vi "ScriptAllClasses.vi"(8 "error in (no error)":errorcluster, 11 "Application in":refnum<class "Application.lvclass">) -> (0 "error out":errorcluster, 3 "Application out":refnum<class "Application.lvclass">)   [LabVIEW 2020, in "Mermaid.lvlib" / "Application.lvclass"]
uses:
  Application.lvclass
  Application.lvclass/Application.ctl
  _Class/Class.lvclass
  _Interface/Interface.lvclass
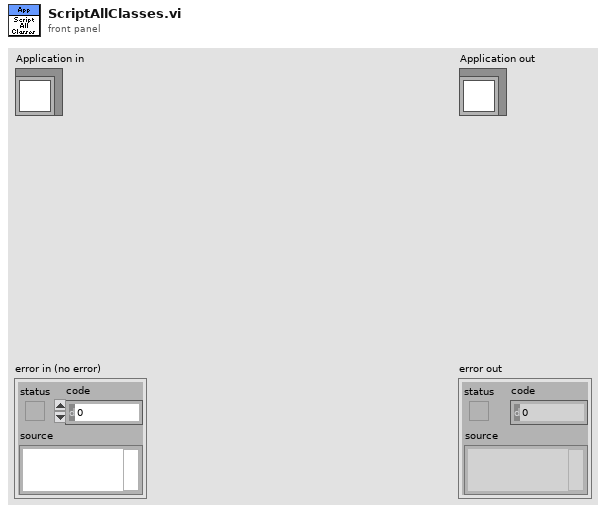
[diagram p1: front panel]
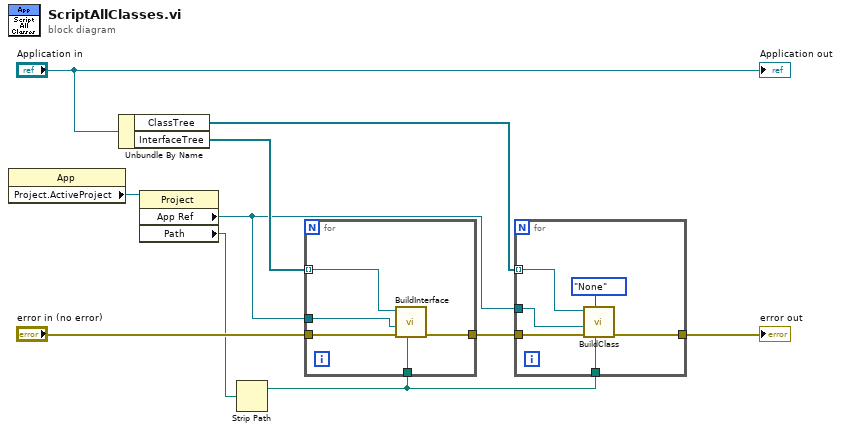
[diagram p0: block diagram]
diagram:
  n1 = property class="App"() -> ("Project.ActiveProject"=w5:refnum<vi>)  [unwired: 2 in, 2 out]
  n2 = Unbundle By Name("Application in") -> ("ClassTree"=w7:refnum<class "Class.lvclass">[], "InterfaceTree"=w9:refnum<class "Interface.lvclass">[])
  n3 = property class="Project"(reference=w5) -> ("App Ref"=w3:refnum<vi>, "Path"=w2:path)  [unwired: 1 in, 2 out]
  n4 = Strip Path(path=w2) -> (stripped path=w1:path)  [unwired: 1 out]
  n5 = for {
    tunnel: w9 -> [w15] mode=indexing
    tunnel: w3 -> [w12]
    tunnel: "error in (no error)" -> [w14]
    tunnel: [w13] -> w4
    tunnel: w1 -> [w11]
    n6 = call "BuildInterface.vi"("ProjectPath"=w11, "error in (no error)"=w14, "Application"=w12, "Interface in"=w15) -> ("error out"=w13:errorcluster)  [unwired: 6 in, 1 out]
  }
  n7 = for {
    tunnel: w7 -> [w18] mode=indexing
    tunnel: w4 -> [w21]
    tunnel: [w20] -> w6
    tunnel: w3 -> [w19]
    tunnel: w1 -> [w16]
    n8 = call-dynamic "BuildClass.vi"("ProjectPath"=w16, "Parent"=enum16{"None", "Interface", "Class"}."None", "error in (no error)"=w21, "Application"=w19, "Class in"=w18) -> ("error out"=w20:errorcluster)  [unwired: 5 in, 1 out]
  }
  "error out" <- w6
  "Application out" <- "Application in"
